vi "GetInputTypeString.vi"(7 "DLL path":path, 8 "error in (no error)":errorcluster, 10 "input Index":i32, 11 "session id in":i32) -> (0 "error out":errorcluster, 1 "InputTypeName":string, 3 "session id out":i32)   [LabVIEW 2017, in "ONNX Class Library.lvlib"]
doc: "/**\n * @brief Получить имя типа данных входа в виде строки\n * \n * Возвращает человекочитаемое имя типа данных (например, \"FLOAT32\", \"INT64\").\n * Удобно для отображения в интерфейсе LabVIEW и логирования.\n * \n * @param sessionId [IN] ID сессии\n * @param inputIndex [IN] Индекс входа (0-based)\n * @param buffer [OUT] Буфер для строки с именем типа\n * @param bufferSize [IN] Размер буфера в байтах (рекомендуется 32 или больше)\n * \n * @return int32: 0 при успешном копировании имени типа\n * @return int32: -1 если сессия не найдена или индекс неверен\n * \n * @note Возможные значения: \"FLOAT32\", \"FLOAT64\", \"INT8\", \"INT16\", \"INT32\", \n * \"INT64\", \"UINT8\", \"UINT16\", \"UINT32\", \"UINT64\", \"FLOAT16\", \"UNKNOWN\"\n */\nint GetInputTypeString(int sessionId, int inputIndex, char* buffer, int bufferSize);"
uses:
  ONNX Class Library.lvlib
panel:
  out "bufferSize":i32
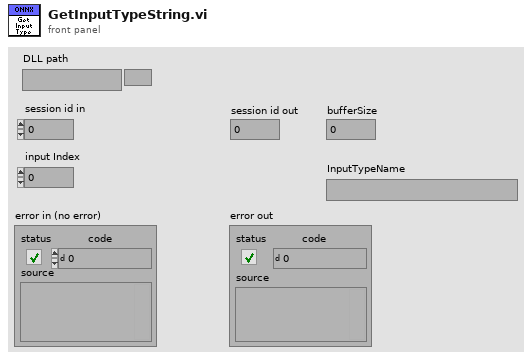
[diagram p1: front panel]
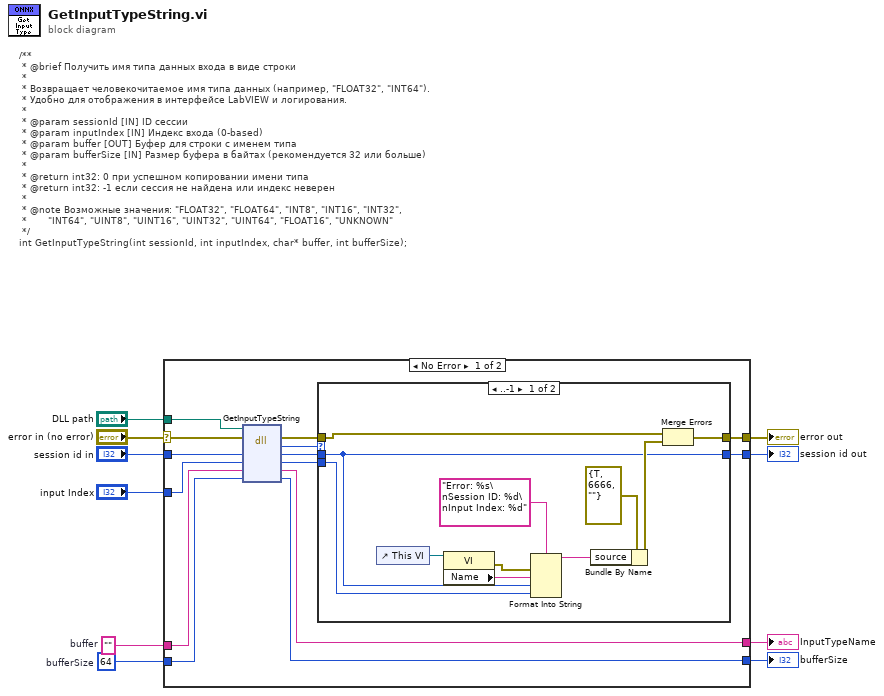
[diagram p0: block diagram]
diagram:
  w7 = 64  # bufferSize
  w9 = ""  # buffer
  # "/**\n * @brief Получить имя типа данных входа в виде строки\n * \n * Возвращает человекочитаемое имя типа данных (например, \"FLOAT32\", \"INT64\").\n * Удобно для отображения в интерфейсе LabVIEW и логирования.\n * \n * @param sessionId [IN] ID сессии\n * @param inputIndex [IN] Индекс входа (0-based)\n * @param buffer [OUT] Буфер для строки с именем типа\n * @param bufferSize [IN] Размер буфера в байтах (рекомендуется 32 или больше)\n * \n * @return int32: 0 при успешном копировании имени типа\n * @return int32: -1 если сессия не найдена или индекс неверен\n * \n * @note Возможные значения: \"FLOAT32\", \"FLOAT64\", \"INT8\", \"INT16\", \"INT32\", \n *       \"INT64\", \"UINT8\", \"UINT16\", \"UINT32\", \"UINT64\", \"FLOAT16\", \"UNKNOWN\"\n */\nint GetInputTypeString(int sessionId, int inputIndex, char* buffer, int bufferSize);"
  n1 = case shown="No Error" "error in (no error)" {
    selector: "error in (no error)" -> [w11 w39]
    tunnel: "input Index" -> [w24 _]
    tunnel: w9 -> [w23 _]
    tunnel: [w22 _] -> w8
    tunnel: w7 -> [w21 _]
    tunnel: "session id in" -> [w20 w38]
    tunnel: [w19 _] -> w5
    tunnel: [w14 w39] -> w4
    tunnel: [w13 w38] -> w3
    tunnel: "DLL path" -> [w12 _]
    frame No Error {
      n2 = dll-call lib="home/ivan/LabVIEWData/ONNX/Test/libonnx_wrapper/unix64/libonnx_wrapper.so" fn="GetInputTypeString"(path in=w12, error in=w11, "sessionId"=w20, "inputIndex"=w24, "buffer"=w23, "bufferSize"=w21) -> (error out=w18:errorcluster, "return"=w17:i32, "sessionId"=w16:i32, "inputIndex"=w15:i32, "buffer"=w22:string, "bufferSize"=w19:i32)  [unwired: 1 in, 1 out]
      n3 = case shown="..-1" w17 {
        tunnel: w18 -> [w26 w37]
        tunnel: [w27 w37] -> w14
        tunnel: w16 -> [w28 w36]
        tunnel: [w28 w36] -> w13
        tunnel: w15 -> [w25 _]
        frame ..-1 {
          n4 = control-ref of="This VI"() -> (w32:refnum<vi>)
          n5 = property class="VI"(reference=w32) -> (error out=w29:errorcluster, "Name"=w31:string)  [unwired: 1 in, 1 out]
          n6 = Format Into String(format string="Error: %s\nSession ID: %d\nInput Index: %d", error in=w29, w31, w28, w25) -> (resulting string=w33:string)  [unwired: 1 in, 1 out]
          n7 = Bundle By Name(cluster=errorcluster {"status"=TRUE, "code"=6666, "source"=""} ("error out"), "source"=w33) -> (w34:errorcluster)
          n8 = Merge Errors(w26, w34) -> (w27:errorcluster)
        }
        frame 0.. {
        }
      }
    }
    frame Error {
    }
  }
  "error out" <- w4
  "session id out" <- w3
  "InputTypeName" <- w8
  "bufferSize" <- w5
